vi "Edit MATLAB File.vi"() -> ()   [LabVIEW 2020]
panel:
  out "Output":dbl
  in  "B":dbl
  in  "A":dbl
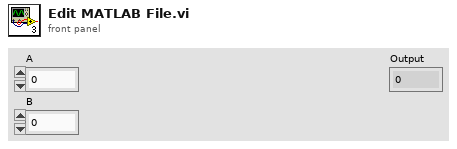
[diagram p1: front panel]
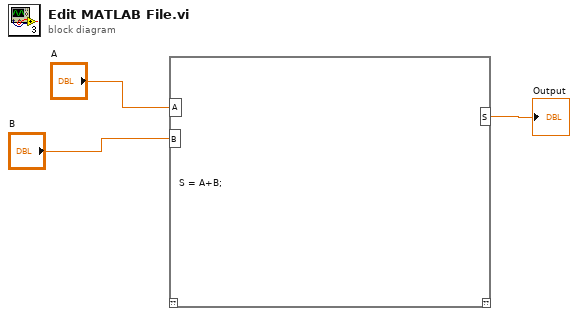
[diagram p0: block diagram]
diagram:
  n1 = script code="S = A+B;"("A"="A", "B"="B") -> ("S"=→"Output":dbl)  [unwired: 1 in, 1 out]
